vi "AMI_Split_Cluster.vi"(0 "AMI_Cluster":T3={"Set Persistent"=FALSE, "B (T)"=1.0, "B Setpoint (T)"=0.0, "Phi (Deg)"=0.0, "Phi Setpoint (Deg)"=0.0, "B Rate (T/min)"=0.0, "Y-Axis (T)"=0.0, "Z-Axis (T)"=0.0, "Z-Axis State"=enum."", "Y-Axis State"=enum."RAMPING", "Update"=FALSE, "Persistent?"=FALSE}) -> (1 "AMI_Status":T2={"Y-Axis (T)"=0.0, "Z-Axis (T)"=0.0, "B AMI (T)"=0.0, "Phi (Deg) "=0.0, "Persistent?"=FALSE, "Z-Axis State"=enum."RAMPING", "Y-Axis State"=enum."RAMPING"}, 2 "AMI_Control":T1)   [LabVIEW 2019]
uses:
  AMI/AMI_cluster.ctl
  AMI/AMI_Status.ctl
  AMI/AMI_Control.ctl
panel:
  # "AMI-Cluster"
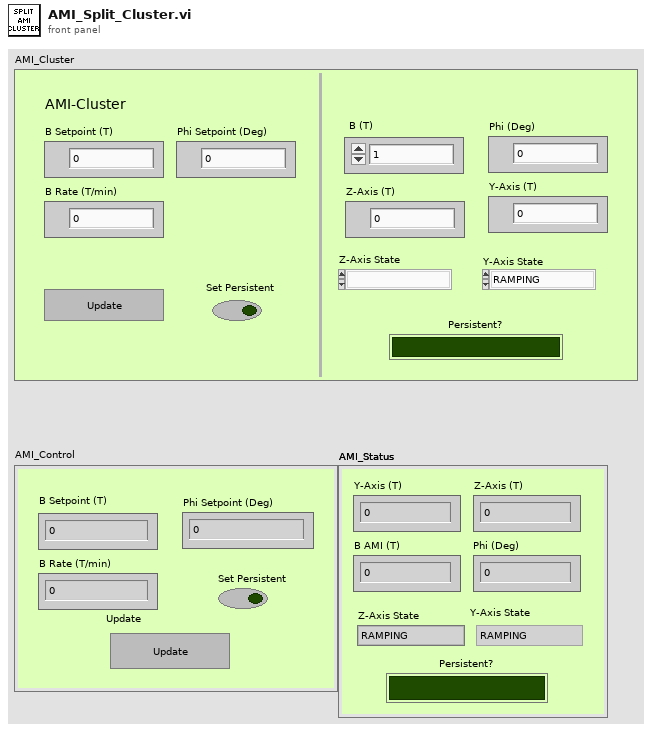
[diagram p1: front panel]
types:
  T1 = typedef "AMI_Control.ctl" = cluster{"B Rate (T/min)":dbl, "B Setpoint (T)":dbl, "Phi Setpoint (Deg)":dbl, "Set Persistent":bool, "Update":bool}
  T2 = typedef "AMI_Status.ctl" = cluster{"Y-Axis (T)":dbl, "Z-Axis (T)":dbl, "B AMI (T)":dbl, "Phi (Deg) ":dbl, "Persistent?":bool, "Z-Axis State":enum16{"", "RAMPING", "HOLDING", "PAUSED", "MANUAL UP", "MANUAL DOWN", "ZEROING CURRENT", "QUENCH DETECTED", "AT ZERO", "HEATING SWITCH", "COOLING SWITCH", "EXTERNAL RAMPDOWN"}, "Y-Axis State":enum16{"", "RAMPING", "HOLDING", "PAUSED", "MANUAL UP", "MANUAL DOWN", "ZEROING CURRENT", "QUENCH DETECTED", "AT ZERO", "HEATING SWITCH", "COOLING SWITCH", "EXTERNAL RAMPDOWN"}}
  T3 = typedef "AMI_cluster.ctl" = cluster{"Set Persistent":bool, "B (T)":dbl, "B Setpoint (T)":dbl, "Phi (Deg)":dbl, "Phi Setpoint (Deg)":dbl, "B Rate (T/min)":dbl, "Y-Axis (T)":dbl, "Z-Axis (T)":dbl, "Z-Axis State":enum16{"", "RAMPING", "HOLDING", "PAUSED", "MANUAL UP", "MANUAL DOWN", "ZEROING CURRENT", "QUENCH DETECTED", "AT ZERO", "HEATING SWITCH", "COOLING SWITCH", "EXTERNAL RAMPDOWN"}, "Y-Axis State":enum16{"", "RAMPING", "HOLDING", "PAUSED", "MANUAL UP", "MANUAL DOWN", "ZEROING CURRENT", "QUENCH DETECTED", "AT ZERO", "HEATING SWITCH", "COOLING SWITCH", "EXTERNAL RAMPDOWN"}, "Update":bool, "Persistent?":bool}
  T4 = enum16{"", "RAMPING", "HOLDING", "PAUSED", "MANUAL UP", "MANUAL DOWN", "ZEROING CURRENT", "QUENCH DETECTED", "AT ZERO", "HEATING SWITCH", "COOLING SWITCH", "EXTERNAL RAMPDOWN"}
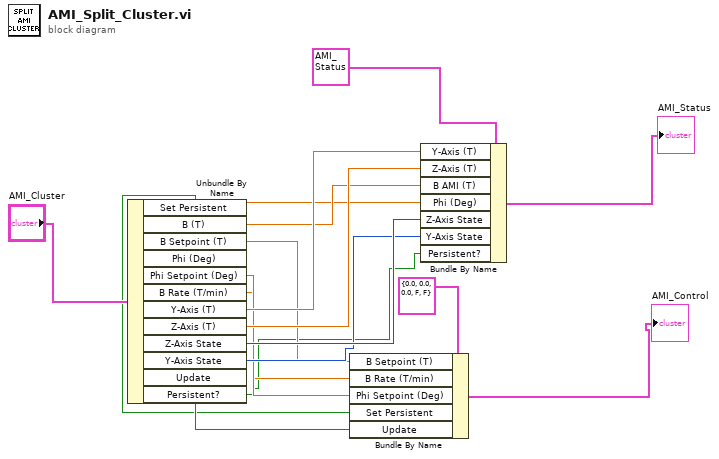
[diagram p0: block diagram]
diagram:
  n1 = Unbundle By Name("AMI_Cluster") -> ("Set Persistent"=w1:bool, "B (T)"=w10:dbl, "B Setpoint (T)"=w6:dbl, "Phi (Deg)"=w9:dbl, "Phi Setpoint (Deg)"=w5:dbl, "B Rate (T/min)"=w4:dbl, "Y-Axis (T)"=w12:dbl, "Z-Axis (T)"=w11:dbl, "Z-Axis State"=w8:T4, "Y-Axis State"=w7:T4, "Update"=w3:bool, "Persistent?"=w2:bool)
  n2 = Bundle By Name(cluster=T1 {"B Rate (T/min)"=0.0, "B Setpoint (T)"=0.0, "Phi Setpoint (Deg)"=0.0, "Set Persistent"=FALSE, "Update"=FALSE} ("AMI_Control 2"), "B Setpoint (T)"=w6, "B Rate (T/min)"=w4, "Phi Setpoint (Deg)"=w5, "Set Persistent"=w1, "Update"=w3) -> (→"AMI_Control":T1)
  n3 = Bundle By Name(cluster=T2 {"Y-Axis (T)"=0.0, "Z-Axis (T)"=0.0, "B AMI (T)"=0.0, "Phi (Deg) "=0.0, "Persistent?"=FALSE, "Z-Axis State"=enum."RAMPING", "Y-Axis State"=enum."RAMPING"} ("AMI_Status 2"), "Y-Axis (T)"=w12, "Z-Axis (T)"=w11, "B AMI (T)"=w10, "Phi (Deg)"=w9, "Z-Axis State"=w8, "Y-Axis State"=w7, "Persistent?"=w2) -> (→"AMI_Status":T2)
